vi "运控模式参数配置.vi"(1 "Kd":dbl(slide) scale=0.0..5.0 scale format="%#_4g", 2 "电机ID":string, 3 "Kp":dbl(slide) scale=0.0..500.0, 4 "速度":dbl(slide) scale=-30.0..30.0, 5 "扭矩":dbl(slide) scale=-12.0..12.0, 6 "位置":dbl(slide) scale=-12.5..12.5) -> (0 "最终输出报文":string)   [LabVIEW 2023]
panel:
  out "输出位置报文":string
  out "输出角速度报文":string
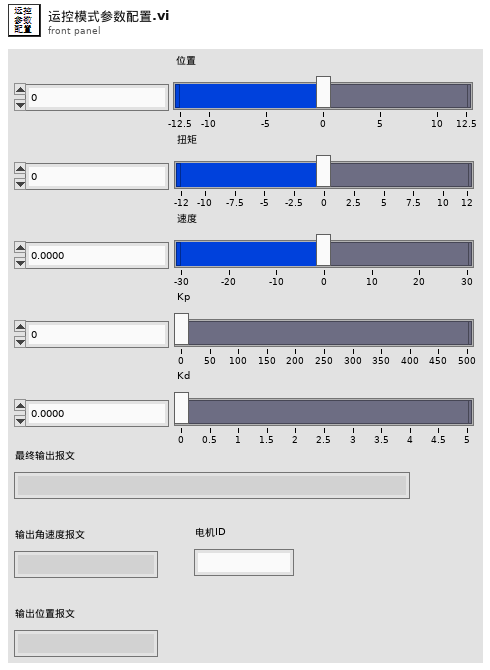
[diagram p1: front panel]
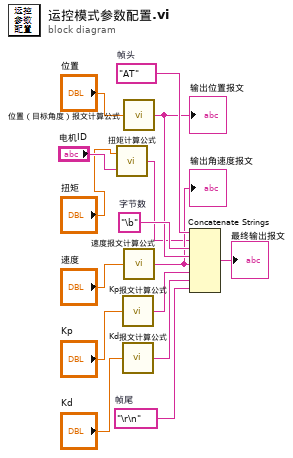
[diagram p0: block diagram]
diagram:
  w8 = "\r\n"  # 帧尾
  w15 = "\b"  # 字节数
  w14 = "AT"  # 帧头
  n1 = call "扭矩计算公式.vi"("电机ID"="电机ID", "扭矩"="扭矩") -> ("最终输出报文 2"=w1:string)
  n2 = call "Kp报文计算公式.vi"("Kp"="Kp") -> ("Kp报文"=w7:string)
  n3 = call "Kd报文计算公式.vi"("Kd"="Kd") -> ("Kd报文"=w5:string)
  n4 = call "位置（目标角度）报文计算公式.vi"("位置"="位置") -> ("输出位置报文"=w11:string)
  "输出位置报文" <- w11
  n5 = call "速度报文计算公式.vi"("速度"="速度") -> ("输出角速度报文"=w10:string)
  "输出角速度报文" <- w10
  n6 = Concatenate Strings(w14, w1, w15, w11, w10, w7, w5, w8) -> (→"最终输出报文":string)
